vi "Using the State Machine Architecture.vi"() -> ()   [LabVIEW 2020]
uses:
  status.ctl
  computer hand.ctl
  main cases.ctl
  Creating an Action Engine/timer states.ctl
panel:
  in  "Exit Button":bool
  in  "Scissors Button":bool
  in  "Paper Button":bool
  in  "Rock Button":bool
  out "Computer Hand":T1=enum."Blank"
  out "Status":T2=enum."You Lose!!!"
  in  "Reset":bool
  in  "Start":bool
  out "error out":errorcluster
  in  "error in":errorcluster
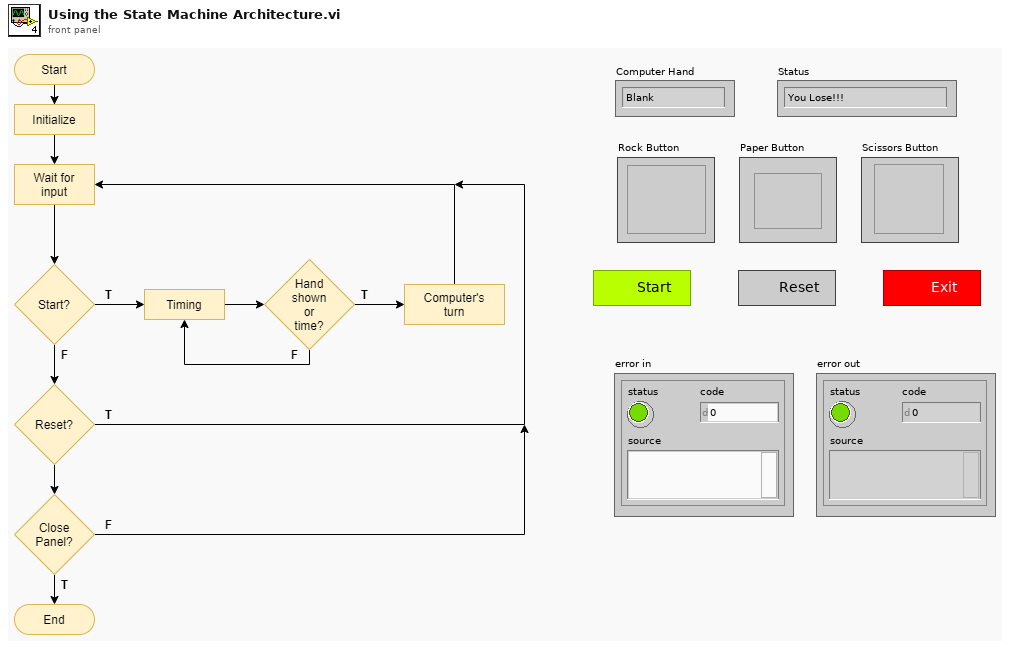
[diagram p1: front panel]
types:
  T1 = typedef "computer hand.ctl" = enum16{"Rock", "Paper", "Scissors", "Blank"}
  T2 = typedef "status.ctl" = enum16{"Click Start to Play!!!", "You Win!!!", "You Lose!!!", "Tie!!!", "1", "2", "GO!!!"}
  T3 = typedef "main cases.ctl" = enum16{"INITIALIZE", "WAIT FOR INPUT", "TIMING", "COMPUTER'S TURN", "SHUTDOWN"}
  T4 = typedef "timer states.ctl" = enum16{"START TIMER", "RESTART TIMER", "CHECK TIMER", "PAUSE TIMER"}
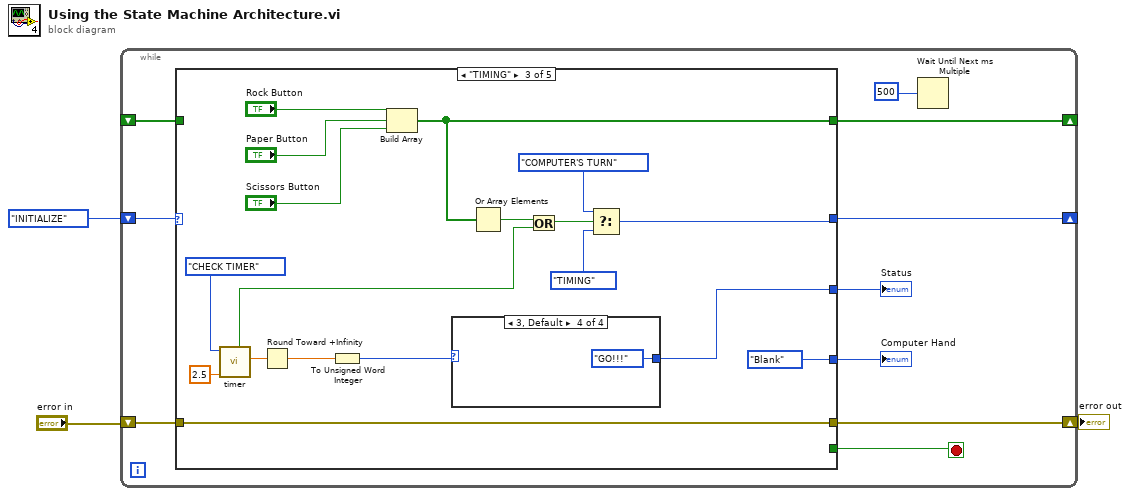
[diagram p0: block diagram]
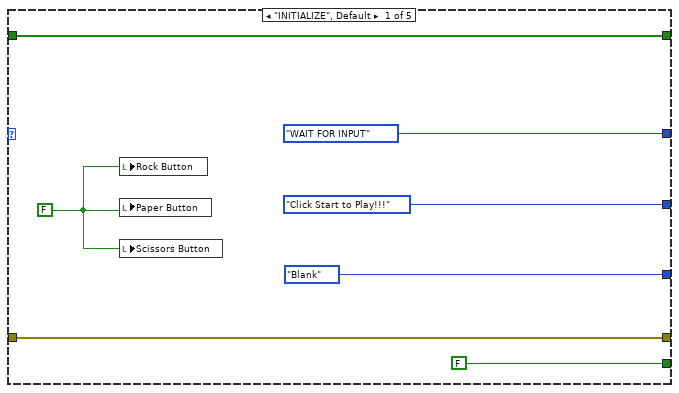
[diagram p2: hidden frame]
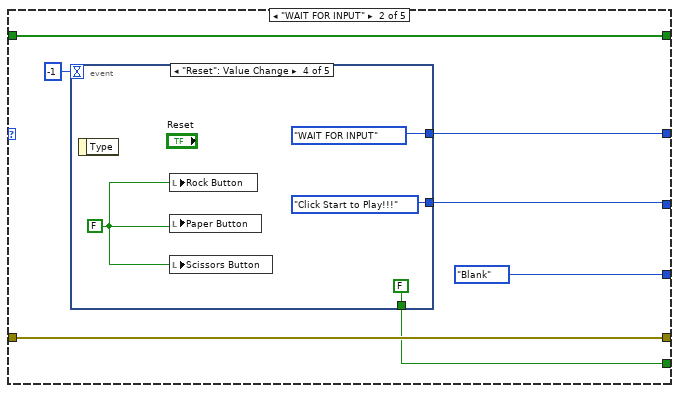
[diagram p3: hidden frame]
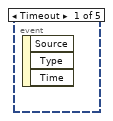
[diagram p4: hidden frame]
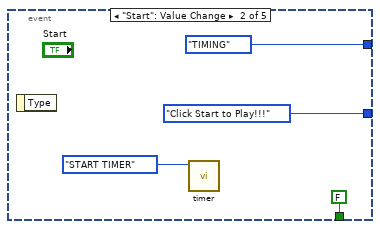
[diagram p5: hidden frame]
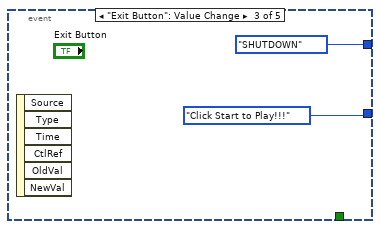
[diagram p6: hidden frame]
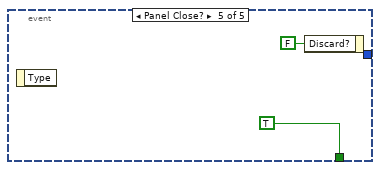
[diagram p7: hidden frame]
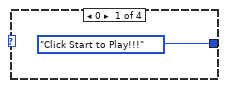
[diagram p8: hidden frame]
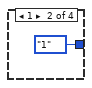
[diagram p9: hidden frame]
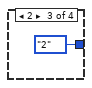
[diagram p10: hidden frame]
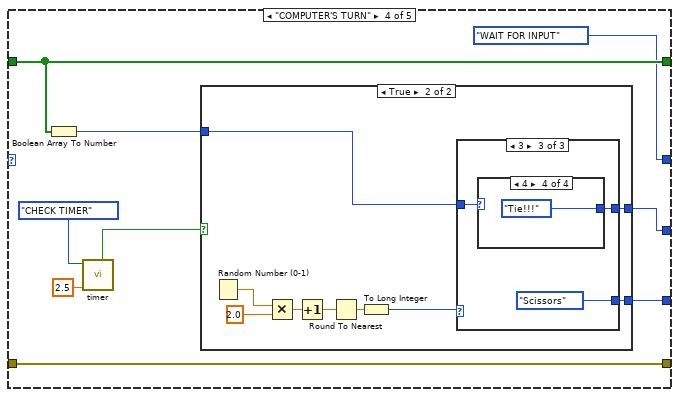
[diagram p11: hidden frame]
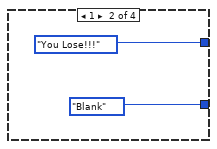
[diagram p13: hidden frame]
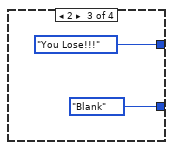
[diagram p14: hidden frame]
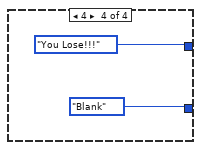
[diagram p15: hidden frame]
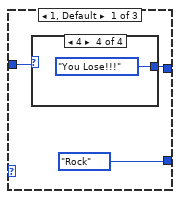
[diagram p16: hidden frame]
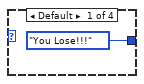
[diagram p17: hidden frame]
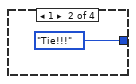
[diagram p18: hidden frame]
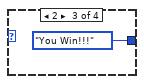
[diagram p19: hidden frame]
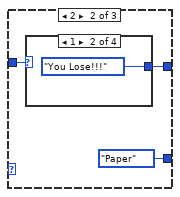
[diagram p20: hidden frame]
diagram:
  n1 = while {
    shift-right: [w12] -> _
    shift-left: _ -> [w11]
    shift-right: [w6] -> _
    shift-left: main_cases."INITIALIZE" -> [w13]
    shift-right: [w9] -> w2
    shift-left: "error in" -> [w10]
    stop <- w8 stop-if-true
    n2 = case shown="\"TIMING\"" w13 {
      tunnel: [w20 w27 w52 w70 _] -> w12
      tunnel: w11 -> [w20 w27 _ w70 _]
      tunnel: [w19 w26 w42 w66 _] -> w9
      tunnel: w10 -> [w19 w26 w42 w66 _]
      tunnel: [FALSE w21 _ _ TRUE] -> w8
      tunnel: [main_cases."WAIT FOR INPUT" w24 w49 main_cases."WAIT FOR INPUT" _] -> w6
      tunnel: [status."Click Start to Play!!!" w23 w44 w64 _] -> w5
      tunnel: [computer_hand."Blank" computer_hand."Blank" computer_hand."Blank" w63 _] -> w4
      frame "INITIALIZE", Default {
        w14 = FALSE
        n3 = local write "Rock Button"(w14) -> ()
        n4 = local write "Paper Button"(w14) -> ()
        n5 = local write "Scissors Button"(w14) -> ()
      }
      frame "WAIT FOR INPUT" {
        n6 = event shown="[3] \"Reset\": Value Change" {
          selector: _ -> [_ _ _ _ _]
          dyn-events: _ -> [_ _ _ _ _]
          timeout: -1 -> [_ _ _ _ _]
          tunnel: [_ main_cases."TIMING" main_cases."SHUTDOWN" main_cases."WAIT FOR INPUT" _] -> w24
          tunnel: [_ status."Click Start to Play!!!" status."Click Start to Play!!!" status."Click Start to Play!!!" _] -> w23
          tunnel: [_ FALSE _ FALSE TRUE] -> w21
          event Timeout {
            n7 = event-data() -> ()  [unwired: 1 in, 3 out]
          }
          event "Start": Value Change {
            n8 = event-data() -> ()  [unwired: 1 in, 1 out]
            n9 = call "timer.vi"("Enum"=timer_states."START TIMER") -> ()  [unwired: 9 in, 2 out]
          }
          event "Exit Button": Value Change {
            n10 = event-data() -> ()  [unwired: 1 in, 6 out]
          }
          event "Reset": Value Change {
            w35 = FALSE
            n11 = event-data() -> ()  [unwired: 1 in, 1 out]
            n12 = local write "Rock Button"(w35) -> ()
            n13 = local write "Paper Button"(w35) -> ()
            n14 = local write "Scissors Button"(w35) -> ()
          }
          event Panel Close? {
            n15 = event-data() -> ()  [unwired: 1 in, 1 out]
            n16 = event-data("Discard?"=FALSE) -> ()  [unwired: 1 in, 1 out]
          }
        }
      }
      frame "TIMING" {
        n17 = call "timer.vi"("Time Duration"=2.5, "Enum"=timer_states."CHECK TIMER") -> ("Time Elapsed"=w40:dbl, "Time Elapsed?"=w43:bool)  [unwired: 8 in]
        n18 = Round Toward +Infinity(x=w40) -> (ceil(x): smallest int >= x=w41:dbl)
        n19 = To Unsigned Word Integer(number=w41) -> (unsigned 16bit integer=w45:u16)
        n20 = Build Array "Build Array"("Rock Button", "Paper Button", "Scissors Button") -> (w52:bool[])
        n21 = case shown="3, Default" w45 {
          tunnel: [status."Click Start to Play!!!" status."1" status."2" status."GO!!!"] -> w44
          frame 0 {
          }
          frame 1 {
          }
          frame 2 {
          }
          frame 3, Default {
          }
        }
        n22 = Or Array Elements(Boolean array=w52) -> (logical OR=w53:bool)
        n23 = Or(x=w53, y=w43) -> (x .or. y?=w54:bool)
        n24 = Select(t=main_cases."COMPUTER'S TURN", s=w54, f=main_cases."TIMING") -> (s? t:f=w49:T3)
      }
      frame "COMPUTER'S TURN" {
        n25 = Boolean Array To Number(Boolean array=w70) -> (number=w65:u32)
        n26 = call "timer.vi"("Time Duration"=2.5, "Enum"=timer_states."CHECK TIMER") -> ("Time Elapsed?"=w67:bool)  [unwired: 8 in, 1 out]
        n27 = case shown="True" w67 {
          tunnel: w65 -> [w73 w82]
          tunnel: [w72 w81] -> w64
          tunnel: [w71 w80] -> w63
          frame False {
            n28 = case shown="Default" w73 {
              tunnel: [_ status."You Lose!!!" status."You Lose!!!" status."You Lose!!!"] -> w72
              tunnel: [_ computer_hand."Blank" computer_hand."Blank" computer_hand."Blank"] -> w71
              frame Default {
              }
              frame 1 {
              }
              frame 2 {
              }
              frame 4 {
              }
            }
          }
          frame True {
            n29 = Random Number (0-1)() -> (number: 0 to 1=w87:dbl)
            n30 = Multiply(x=w87, y=2.0) -> (x*y=w86:dbl)
            n31 = Increment(x=w86) -> (x+1=w85:dbl)
            n32 = Round To Nearest(number=w85) -> (nearest integer value=w84:dbl)
            n33 = To Long Integer(number=w84) -> (32bit integer=w83:i32)
            n34 = case shown="3" w83 {
              tunnel: w82 -> [w89 w96 w104]
              tunnel: [w90 w97 w103] -> w81
              tunnel: [computer_hand."Rock" computer_hand."Paper" computer_hand."Scissors"] -> w80
              frame 1, Default {
                n35 = case shown="4" w89 {
                  tunnel: [status."You Lose!!!" status."Tie!!!" status."You Win!!!" status."You Lose!!!"] -> w90
                  frame Default {
                  }
                  frame 1 {
                  }
                  frame 2 {
                  }
                  frame 4 {
                  }
                }
              }
              frame 2 {
                n36 = case shown="1" w96 {
                  tunnel: [status."You Lose!!!" status."You Lose!!!" status."Tie!!!" status."You Win!!!"] -> w97
                  frame Default {
                  }
                  frame 1 {
                  }
                  frame 2 {
                  }
                  frame 4 {
                  }
                }
              }
              frame 3 {
                n37 = case shown="4" w104 {
                  tunnel: [status."You Lose!!!" status."You Win!!!" status."You Lose!!!" status."Tie!!!"] -> w103
                  frame Default {
                  }
                  frame 1 {
                  }
                  frame 2 {
                  }
                  frame 4 {
                  }
                }
              }
            }
          }
        }
      }
      frame "SHUTDOWN" {
      }
    }
    "Status" <- w5
    "Computer Hand" <- w4
    n38 = Wait Until Next ms Multiple(millisecond multiple=u32 500) -> ()  [unwired: 1 out]
  }
  "error out" <- w2
